vi "get_AgentDestination.vi"(8 "error in (no error)":errorcluster, 11 "MoAgSy_Visitor_travel.lvclass in":refnum<class "MoAgSy_Visitor_travel.lvclass">) -> (0 "error out":errorcluster, 2 "destination":string, 3 "MoAgSy_Visitor_travel.lvclass out":refnum<class "MoAgSy_Visitor_travel.lvclass">)   [LabVIEW 2009, in "MoAgSy.lvlib" / "MoAgSy_Visitor_travel.lvclass"]
doc: "returns the destination attribute to set agents travel destination"
uses:
  MoAgSy_Visitor_travel.lvclass
  MoAgSy_Visitor_travel.lvclass/MoAgSy_Visitor_travel.ctl
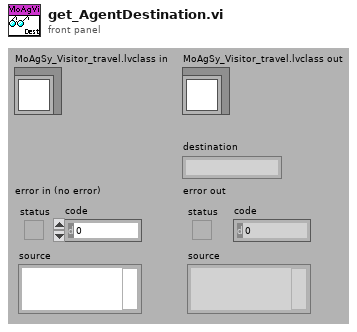
[diagram p1: front panel]
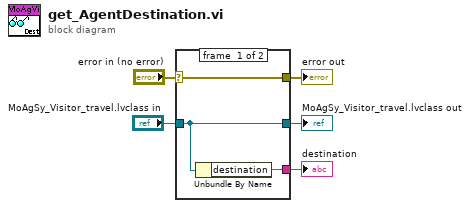
[diagram p0: block diagram]
diagram:
  n1 = case shown="No Error" "error in (no error)" {
    selector: "error in (no error)" -> [w8 w9]
    tunnel: [w8 w9] -> w4
    tunnel: [w7 w10] -> w2
    tunnel: "MoAgSy_Visitor_travel.lvclass in" -> [w7 w10]
    tunnel: [w6 _] -> w1
    frame #0 {
      n2 = Unbundle By Name(w7) -> ("destination"=w6:string)
    }
    frame #1 {
    }
  }
  "error out" <- w4
  "MoAgSy_Visitor_travel.lvclass out" <- w2
  "destination" <- w1
